vi "To Waveform.vi"(8 "error in (no error)":errorcluster, 11 "U32 in":refnum<class "U32.lvclass">) -> (0 "error out":errorcluster, 1 "Success?":bool, 3 "Waveform Array":waveform(dbl)[](array[waveform]))   [LabVIEW 2020, in "Data.lvlib" / "U32.lvclass"]
doc: "Interpret 'Data' as a Waveform Array. If impossible 'Success?' is set to FALSE"
uses:
  U32.lvclass
  U32.lvclass/U32.ctl
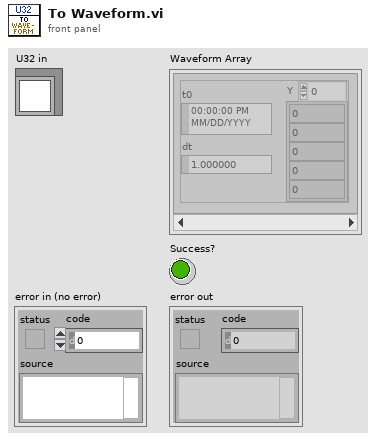
[diagram p1: front panel]
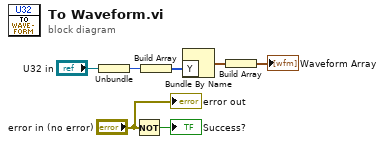
[diagram p0: block diagram]
diagram:
  n1 = Unbundle("U32 in") -> (w6:u32)
  n2 = Not(x="error in (no error)") -> (.not. x?=→"Success?":bool)
  n3 = Build Array(w6) -> (w4:u32[])
  n4 = Bundle By Name("Y"=w4) -> (w7:waveform(u32))  [unwired: 1 in]
  n5 = Build Array(w7) -> (→"Waveform Array":waveform(u32)[])
  "error out" <- "error in (no error)"
